vi "Initialize chart.vi"(4 "Variables":T2) -> (1 "Chart":T1(graph))   [LabVIEW 2020]
uses:
  Constants.ctl
  <resource>/objmgr/daqmx.rc
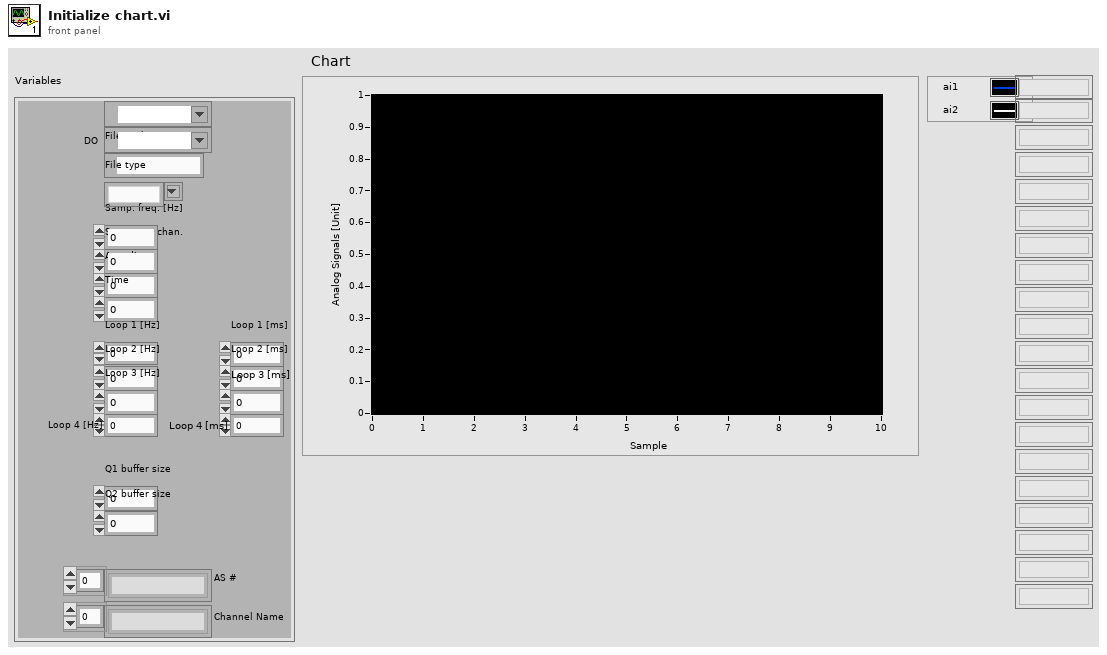
[diagram p1: front panel]
types:
  T1 = cluster{"[0]":dbl, "[1]":dbl, "[2]":dbl, "[3]":dbl, "[4]":dbl, "[5]":dbl, "[6]":dbl, "[7]":dbl, "[8]":dbl, "[9]":dbl, "[10]":dbl, "[11]":dbl, "[12]":dbl, "[13]":dbl, "[14]":dbl, "[15]":dbl, "[16]":dbl, "[17]":dbl, "[18]":dbl, "[19]":dbl}
  T2 = typedef "Constants.ctl" = cluster{"Time":u16, "Samp. freq. [Hz]":dbl, "Samp. per chan.":i32, "Avg. div.":i32, "File path":path, "AI":refnum<k21>, "Loop 1 [Hz]":dbl, "Loop 2 [Hz]":dbl, "Loop 3 [Hz]":dbl, "Loop 1 [ms]":dbl, "Loop 2 [ms]":dbl, "Loop 3 [ms]":dbl, "Q1 buffer size":i32, "Q2 buffer size":i32, "File type":string, "Loop 4 [Hz]":dbl, "Loop 4 [ms]":dbl, "Channel Name":string[], "AS #":string[], "DO":refnum<k21>}
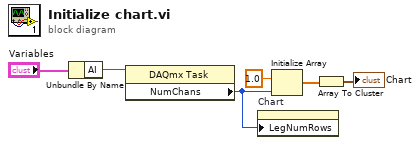
[diagram p0: block diagram]
diagram:
  n1 = Unbundle By Name("Variables") -> ("AI"=w5:refnum<k21>)
  n2 = property class="DAQmx Task"(reference=w5) -> ("NumChans"=w1:u32)  [unwired: 1 in, 2 out]
  n3 = property on="Chart" class="WFChart (strict)"("LegNumRows"=w1) -> ()  [unwired: 2 in, 2 out]
  n4 = Initialize Array(1.0 ("element"), w1) -> (w3:dbl[])
  n5 = Array To Cluster(array=w3) -> (cluster=→"Chart":T1)
